vi "Facade 3.vi"(0 "Data In":T6, 2 "Display State In":T4, 3 "Container State":T5) -> (6 "Data Out":T6, 7 "Display State Out":T4, 8 "Action":T3)   [LabVIEW 2011, in "Criteria control.xctl"]
uses:
  Criteria control.xctl
  Data 3.ctl
  Single criteria cluster.ctl
  Criteria types.ctl
  <vilib>/_xctls/Container State.ctl
  State 3.ctl
  <vilib>/_xctls/Action.ctl
  <vilib>/_xctls/XControlSupport.lvlib
panel:
  in  "Criteria":T1
  out "Tab Control":T2(tab)
  in  "Digital IO":u16(ring)
  in  "Time":dbl caption="Time(s)" format="%#.1f"
  in  "User limit":bool
  in  "Analog IO":u16(ring)
  in  "Analog limit 1":dbl caption="Limit" format="%#_6f"
  in  "Limit analog 2":dbl caption="Limit" format="%#_6f"
  in  "Analog IO 1":u16(ring)
  in  "Analog IO 2":u16(ring)
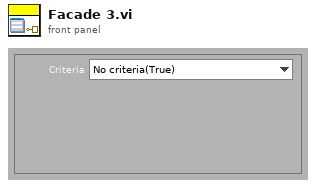
[diagram p1: front panel]
types:
  T1 = typedef "Criteria types.ctl" = enum16{"No criteria(True)", "Time(s)", "Analog IO over", "Analog IO over or equal", "Analog IO under", "Analog IO under or equal", "Analog IO 1 minus Analog IO 2 over", "Digital IO True", "Digital IO False", "Operator approval"}
  T2 = enum32{"Nothing", "One digital", "Time", "One dbl", "Two dbl"}
  T3 = typedef "XControlSupport.lvlib/Action.ctl" = cluster{"Data Changed?":bool, "State Changed?":bool, "Action Name":string}
  T4 = typedef "Criteria control.xctl/State 3.ctl" = cluster{"Analog IO List":string[], "Digital IO List":string[]}
  T5 = typedef "XControlSupport.lvlib/Container State.ctl" = cluster{"Indicator?":bool, "Run Mode?":bool, " Refnum":refnum<vi>}
  T6 = typedef "Criteria control.xctl/Data 3.ctl" = cluster{"Criteria":T7}
  T7 = typedef "Single criteria cluster.ctl" = cluster{"Criteria":T1, "Time or analog value":dbl, "Primary IO index":i32, "Secondary  IO index":i32, "User_input":bool}
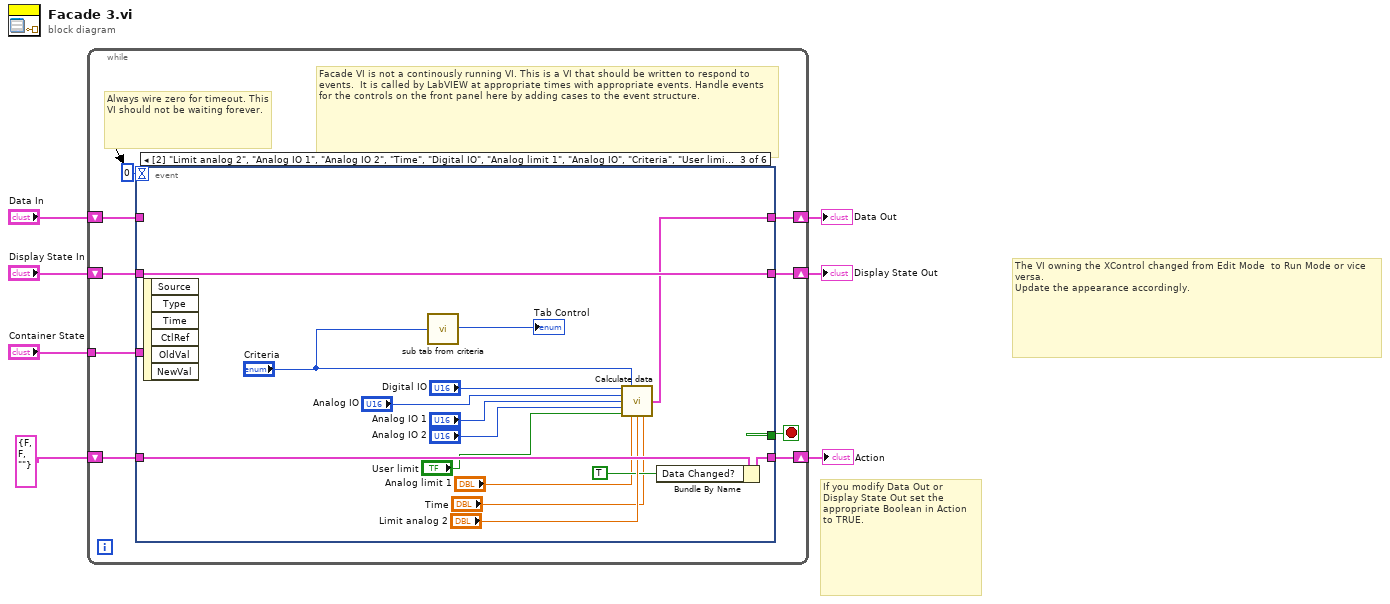
[diagram p0: block diagram]
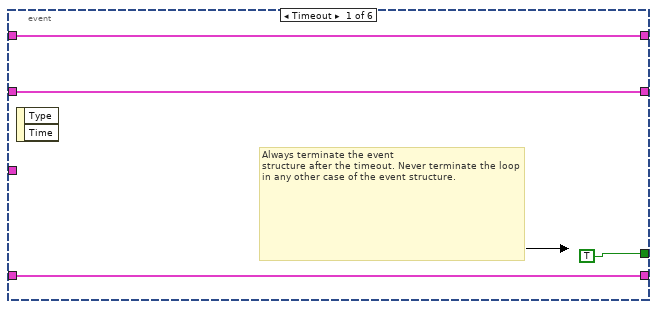
[diagram p2: hidden frame]
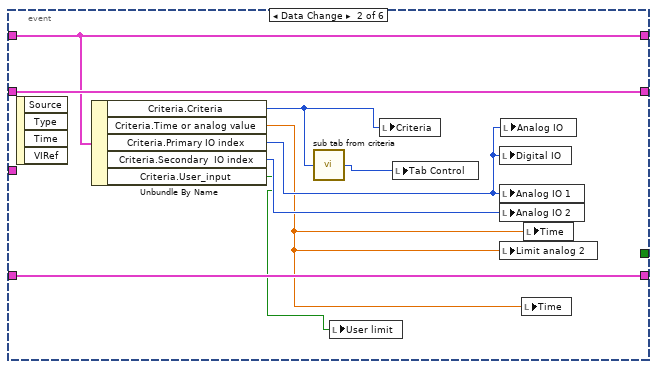
[diagram p3: hidden frame]
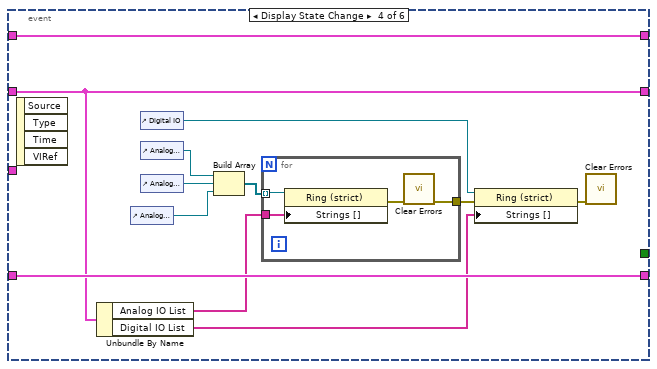
[diagram p4: hidden frame]
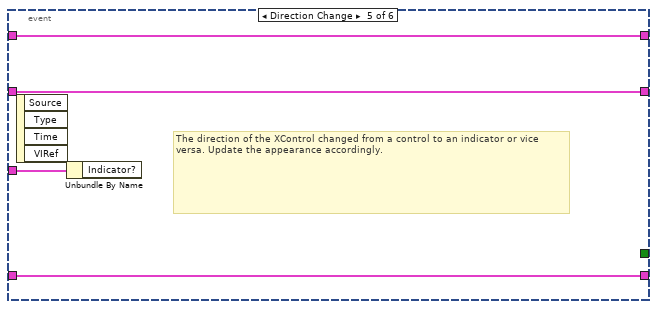
[diagram p5: hidden frame]
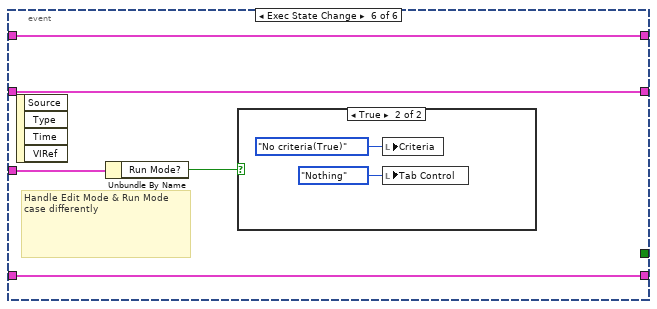
[diagram p6: hidden frame]
diagram:
  # "The VI owning the XControl changed from Edit Mode  to Run Mode or vice versa.\nUpdate the appearance accordingly."
  # "If you modify Data Out or\nDisplay State Out set the\nappropriate Boolean in Action\nto TRUE."
  n1 = while {
    shift-right: [w15] -> w4
    shift-left: "Display State In" -> [w16]
    tunnel: "Container State" -> [w12]
    shift-right: [w10] -> w7
    shift-left: "Data In" -> [w11]
    shift-right: [w8] -> w2
    shift-left: T3 {"Data Changed?"=FALSE, "State Changed?"=FALSE, "Action Name"=""} ("Action") -> [w9]
    stop <- w14 stop-if-true
    # "Facade VI is not a continously running VI. This is a VI that should be written to respond to events.  It is called by LabVIEW at appropriate times with appropriate events. Handle events for the controls on the front panel here by adding cases to the event structure."
    # "Always wire zero for timeout. This\nVI should not be waiting forever."
    n2 = event shown="[2] \"Limit analog 2\", \"Analog IO 1\", \"Analog IO 2\", \"Time\", \"Digital IO\", \"Analog limit 1\", \"Analog IO\", \"Criteria\", \"User limit \": Value Change" {
      selector: _ -> [_ _ _ _ _ _]
      dyn-events: _ -> [_ _ _ _ _ _]
      timeout: 0 -> [_ _ _ _ _ _]
      tunnel: w16 -> [w18 w29 w44 w48 w63 w68]
      tunnel: [w18 w29 w44 w48 w63 w68] -> w15
      tunnel: [TRUE _ _ _ _ _] -> w14
      tunnel: w12 -> [_ _ _ _ w64 w69]
      tunnel: w11 -> [w17 w27 _ w56 w62 w67]
      tunnel: [w17 w27 w42 w56 w62 w67] -> w10
      tunnel: [w19 w28 w35 w55 w61 w65] -> w8
      tunnel: w9 -> [w19 w28 w43 w55 w61 w65]
      event Timeout {
        # "Always terminate the event\nstructure after the timeout. Never terminate the loop in any other case of the event structure."
        n3 = event-data() -> ()  [unwired: 1 in, 2 out]
      }
      event Data Change {
        n4 = event-data() -> ()  [unwired: 1 in, 4 out]
        n5 = Unbundle By Name(w27) -> ("Criteria.Criteria"=w26:T1, "Criteria.Time or analog value"=w22:dbl, "Criteria.Primary IO index"=w23:i32, "Criteria.Secondary  IO index"=w25:i32, "Criteria.User_input"=w21:bool)
        n6 = call "sub tab from criteria.vi"("Criteria"=w26) -> ("Tab Control"=w24:T2)
        n7 = local write "User limit"(w21) -> ()
        n8 = local write "Criteria"(w26) -> ()
        n9 = local write "Tab Control"(w24) -> ()
        n10 = local write "Digital IO"(w23) -> ()
        n11 = local write "Analog IO 1"(w23) -> ()
        n12 = local write "Analog IO 2"(w25) -> ()
        n13 = local write "Limit analog 2"(w22) -> ()
        n14 = local write "Analog IO"(w23) -> ()
        n15 = local write "Time"(w22) -> ()
        n16 = local write "Time"(w22) -> ()
      }
      event "Limit analog 2", "Analog IO 1", "Analog IO 2", "Time", "Digital IO", "Analog limit 1", "Analog IO", "User limit": Value Change {
        n17 = event-data() -> ()  [unwired: 1 in, 6 out]
        n18 = call "sub tab from criteria.vi"("Criteria"="Criteria") -> ("Tab Control"=→"Tab Control":T2)
        n19 = call "Calculate data.vi"("D IO"="Digital IO", "Criteria"="Criteria", "A IO"="Analog IO", "A IO 1"="Analog IO 1", "A IO 2"="Analog IO 2", "Limit in main"="User limit", "Limit analog 1"="Analog limit 1", "Limit analog 2"="Limit analog 2", "Time"="Time") -> ("Data"=w42:T6)  [unwired: 6 in]
        n20 = Bundle By Name(cluster=w43, "Data Changed?"=TRUE) -> (w35:T3)
      }
      event Display State Change {
        n21 = event-data() -> ()  [unwired: 1 in, 4 out]
        n22 = Unbundle By Name(w48) -> ("Analog IO List"=w47:string[], "Digital IO List"=w46:string[])
        n23 = control-ref of="Analog IO"() -> (w45:refnum<vi>)
        n24 = control-ref of="Digital IO"() -> (w51:refnum<vi>)
        n25 = control-ref of="Analog IO 1"() -> (w49:refnum<vi>)
        n26 = control-ref of="Analog IO 2"() -> (w54:refnum<vi>)
        n27 = Build Array(w49, w54, w45) -> (w50:refnum<vi>[])
        n28 = for {
          tunnel: [w59] -> w53
          tunnel: w50 -> [w58] mode=indexing
          tunnel: w47 -> [w57]
          n29 = property class="Ring (strict)"(reference=w58, "Strings []"=w57) -> (error out=w60:errorcluster)  [unwired: 1 in, 1 out]
          n30 = call <vilib>:"Clear Errors.vi"("error in (no error)"=w60) -> ("error out"=w59:errorcluster)  [unwired: 6 in]
        }
        n31 = property class="Ring (strict)"(reference=w51, error in=w53, "Strings []"=w46) -> (error out=w52:errorcluster)  [unwired: 1 out]
        n32 = call <vilib>:"Clear Errors.vi"("error in (no error)"=w52) -> ()  [unwired: 6 in, 1 out]
      }
      event Direction Change {
        # "The direction of the XControl changed from a control to an indicator or vice versa. Update the appearance accordingly."
        n33 = event-data() -> ()  [unwired: 1 in, 4 out]
        n34 = Unbundle By Name(w64) -> ()  [unwired: 1 out]
      }
      event Exec State Change {
        # "Handle Edit Mode & Run Mode\ncase differently"
        n35 = event-data() -> ()  [unwired: 1 in, 4 out]
        n36 = Unbundle By Name(w69) -> ("Run Mode?"=w66:bool)
        n37 = case shown="True" w66 {
          frame False {
          }
          frame True {
            n38 = local write "Criteria"(Criteria_types."No criteria(True)" ("Criteria")) -> ()
            n39 = local write "Tab Control"(T2."Nothing" ("Tab Control")) -> ()
          }
        }
      }
    }
  }
  "Display State Out" <- w4
  "Data Out" <- w7
  "Action" <- w2
